vi "SelectUnitforLoadData.v0.52.vi"(3 "File Contents":string, 4 "File Path":path) -> (0 "Continue?":bool, 1 "WL unit copy":i32(ring)=1 items=["Wavelength", "nm", "eV", "meV", "cm-1"])   [LabVIEW 2025]
doc: "Author: Scott Hannahs <sth@magnet.fsu.edu>\n\nThis software is licensed for use under the “MIT License\"\nCopyright (c) 2025 Scott Hannahs, sth@sth@magnet.sthnet.net\n\nPermission is hereby granted, free of charge, to any person obtaining a copy of this software and associated documentation files (the \"Software\"), to deal in the Software without restriction, including without limitation the rights to use, copy, modify, merge, publish, distribute, sublicense, and/or sell copies of the Software, and to permit persons to whom the Software is furnished to do so, subject to the following conditions: The above copyright notice and this permission notice shall be included in all copies or substantial portions of the Software.\n\nTHE SOFTWARE IS PROVIDED \"AS IS\", WITHOUT WARRANTY OF ANY KIND, EXPRESS OR IMPLIED, INCLUDING BUT NOT LIMITED TO THE WARRANTIES OF MERCHANTABILITY, FITNESS FOR A PARTICULAR PURPOSE AND NONINFRINGEMENT. IN NO EVENT SHALL THE AUTHORS OR COPYRIGHT HOLDERS BE LIABLE FOR ANY CLAIM, DAMAGES OR OTHER LIABILITY, WHETHER IN AN ACTION OF CONTRACT, TORT OR OTHERWISE, ARISING FROM, OUT OF OR IN CONNECTION WITH THE SOFTWARE OR THE USE OR OTHER DEALINGS IN THE SOFTWARE."
panel:
  in  "Cancel":bool
  in  "Continue":bool
  in  "WL unit":i32(ring)=1 items=["Wavelength", "nm", "eV", "meV", "cm-1"]
  # "Please double check the file,\nif it contains valid data, \nselect the wavelength unit \nUSED IN THE FILE:"
  # "Hit \"OK\" to load the data\nor \"Cancel\" to abort."
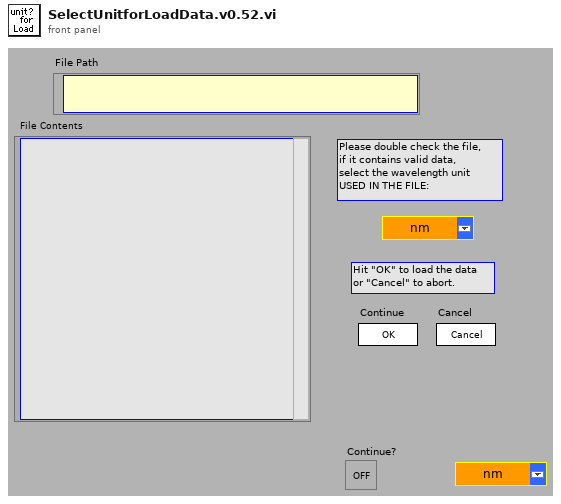
[diagram p1: front panel]
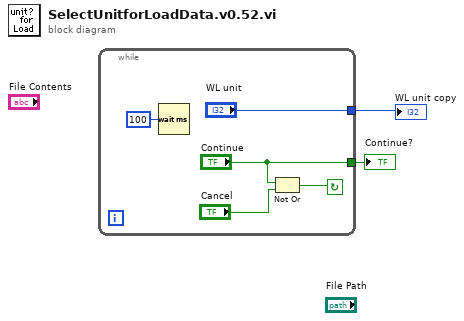
[diagram p0: block diagram]
diagram:
  n1 = while {
    tunnel: ["Continue"] -> w1
    tunnel: ["WL unit"] -> w2
    stop <- w7 continue-if-true
    n2 = Wait (ms)(milliseconds to wait=u32 100) -> ()  [unwired: 1 out]
    n3 = Not Or(1:"Cancel", 2:"Continue") -> (0:w7:bool)
  }
  "WL unit copy" <- w2
  "Continue?" <- w1
